vi "Read_Load_Cell_Tensions.vi"(6 "error in (no error)":errorcluster, 7 "Tare Tension":dbl[](array[numeric])=[1.6875269817998764, 0.7228096971601798, 1.962272927280566, 2.6696462364433735, 2.7003690389898463, 3.088938448864716, 1.6430905755314908, 3.0754139877790347, 3.5546581214666455, 3.2737863413382597, 4.727265898547672, 2.6001067118162604, 1.980007529135911, 1.8614502099489874], 8 "sampling freq [Hz]":dbl=1000.0 format="%#_13g", 9 "Refnum in":refnum<k21>="SCI_TenSen") -> (0 "error out":errorcluster={"status"=TRUE, "code"=-200279, "source"="Read_Load_Cell_Tensions.vi<append>\n<B>Property: </B>RelativeTo\n<B>Requested Value: </B>Current Read Position\n\n<B>Property: </B>Offset\n<B>Requested Value: </B>0\n\n<B>Task Name: </B>SCI_TenSen"}, 2 "Measured Cable Tensions":dbl[](array[numeric])=[nan, nan, nan, nan, nan, nan, nan, nan, nan, nan, nan, nan, nan, nan], 3 "Refnum out":refnum<k21>="SCI_TenSen")   [LabVIEW 2024]
uses:
  <vilib>/Analysis/3filter.llb/Filter Passband Type.ctl
  <vilib>/DAQmx/read.llb/DAQmx Read (Analog 2D DBL NChan NSamp).vi
  <vilib>/Analysis/baseanly.llb/Mean (DBL).vi
  <vilib>/DAQmx/miscellaneous.llb/DAQmx Fill In Error Info.vi
  <vilib>/ptbypt/NI_PtbyPt.lvlib
  <vilib>/Analysis/NI_AALBase.lvlib
panel:
  in  "Load Cell Calibration":dbl[][](array[numeric])=[[124.7777, -0.594, 0.0], [124.887, -0.0754, 0.0], [126.3496, 0.0338, 0.0], [126.1641, 0.0078, 0.0], [122.1693, -0.083, 0.0], [125.7362, 0.3615, 0.0], [124.4104, -0.0707, 0.0], [125.885, -0.4858, 0.0], [124.7524, -0.1227, 0.0], [117.4341, 0.7228, 0.0], [124.1327, 0.2733, 0.0], [125.7391, -0.147, 0.0], [125.9788, -0.1556, 0.0], [123.4595, -0.0054, 0.0], [0.0, 0.0, 124.7777]] format="%#_20g"
  in  "Filter Order":i32=2
  in  "cutoff freq [Hz]":dbl=20.0 format="%0.3f"
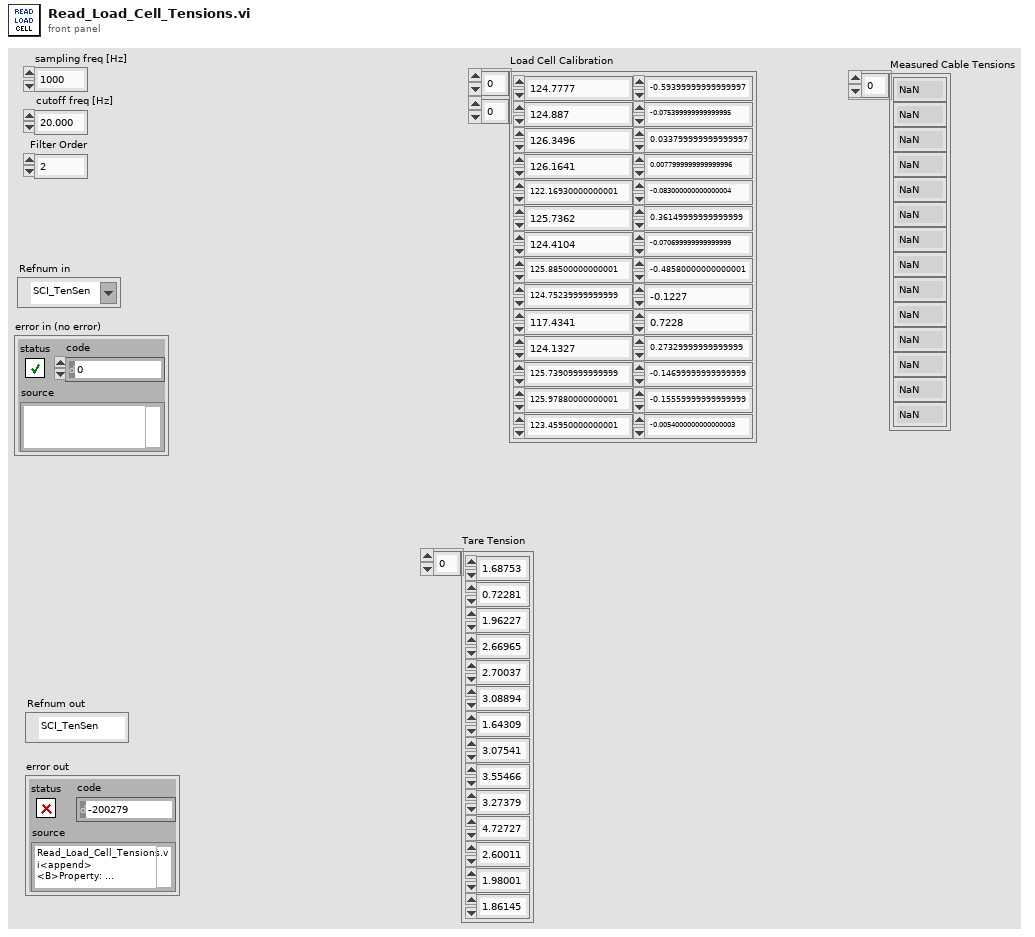
[diagram p1: front panel]
types:
  T1 = typedef "NI_AALBase.lvlib/Filter Passband Type.ctl" = enum32{"Lowpass", "Highpass", "Bandpass", "Bandstop"}
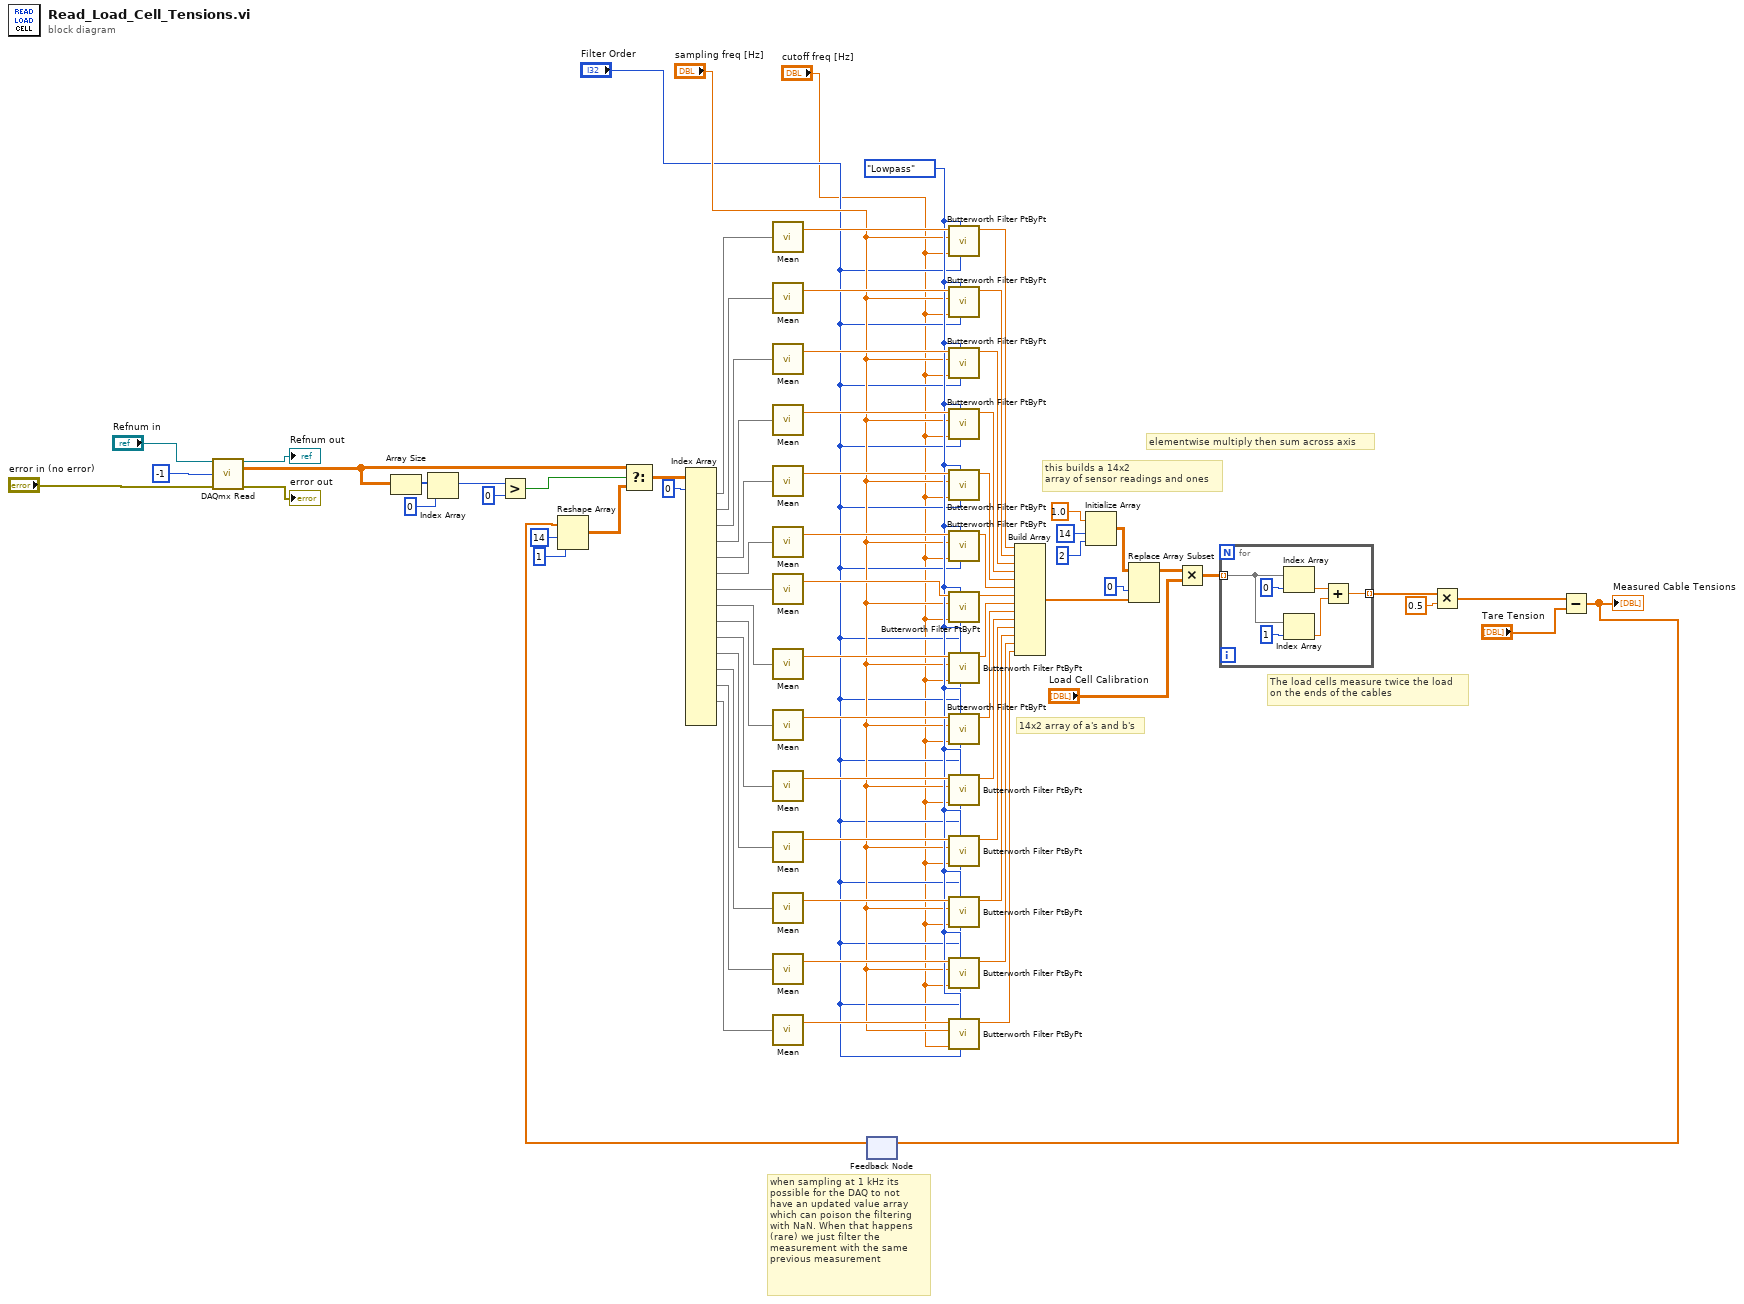
[diagram p0: block diagram]
diagram:
  w14 = Filter_Passband_Type."Lowpass" ("filter type")
  # "when sampling at 1 kHz its \npossible for the DAQ to not\nhave an updated value array\nwhich can poison the filtering\nwith NaN. When that happens\n(rare) we just filter the \nmeasurement with the same\nprevious measurement"
  # "elementwise multiply then sum across axis"
  # "this builds a 14x2\narray of sensor readings and ones"
  # "14x2 array of a's and b's"
  # "The load cells measure twice the load\non the ends of the cables"
  n1 = call-poly <vilib>:"DAQmx Read.vi"("task/channels in"="Refnum in", "number of samples per channel"=-1, "error in"="error in (no error)") -> ("task out"=→"Refnum out":refnum<k21>, "data"=w17:dbl[][], "error out"=→"error out":errorcluster)  [unwired: 10 in]
  n2 = Array Size(array=w17) -> (size(s)=w11:i32[])
  n3 = Index Array(array=w11, index=0) -> (element=w9:i32)
  n4 = Greater?(x=w9, y=0) -> (0:w15:bool)
  n5 = feedback #1() -> (w3:dbl[])  [unwired: 1 in]
  n6 = Reshape Array(w3, 14 ("dimension size"), 1 ("dimension size")) -> (w2:dbl[][])
  n7 = Select(t=w17, s=w15, f=w2) -> (s? t:f=w18:dbl[][])
  n8 = Index Array(array=w18, index (row) #1=0 ("index (row)")) -> (element #1=w57:dbl[], element #2=w68:dbl[], element #3=w67:dbl[], element #4=w66:dbl[], element #5=w65:dbl[], element #6=w64:dbl[], element #7=w63:dbl[], element #8=w60:dbl[], element #9=w48:dbl[], element #10=w47:dbl[], element #11=w46:dbl[], element #12=w45:dbl[], element #13=w44:dbl[], element #14=w43:dbl[])  [unwired: 29 in, 1 out]
  n9 = call-poly <vilib>:"Mean.vi"("X"=w57) -> ("mean"=w56:dbl)  [unwired: 1 out]
  n10 = call-poly <vilib>:"Mean.vi"("X"=w68) -> ("mean"=w74:dbl)  [unwired: 1 out]
  n11 = call-poly <vilib>:"Mean.vi"("X"=w67) -> ("mean"=w73:dbl)  [unwired: 1 out]
  n12 = call-poly <vilib>:"Mean.vi"("X"=w66) -> ("mean"=w72:dbl)  [unwired: 1 out]
  n13 = call-poly <vilib>:"Mean.vi"("X"=w65) -> ("mean"=w71:dbl)  [unwired: 1 out]
  n14 = call-poly <vilib>:"Mean.vi"("X"=w64) -> ("mean"=w70:dbl)  [unwired: 1 out]
  n15 = call-poly <vilib>:"Mean.vi"("X"=w63) -> ("mean"=w69:dbl)  [unwired: 1 out]
  n16 = call-poly <vilib>:"Mean.vi"("X"=w60) -> ("mean"=w59:dbl)  [unwired: 1 out]
  n17 = call-poly <vilib>:"Mean.vi"("X"=w48) -> ("mean"=w42:dbl)  [unwired: 1 out]
  n18 = call-poly <vilib>:"Mean.vi"("X"=w47) -> ("mean"=w41:dbl)  [unwired: 1 out]
  n19 = call-poly <vilib>:"Mean.vi"("X"=w46) -> ("mean"=w40:dbl)  [unwired: 1 out]
  n20 = call-poly <vilib>:"Mean.vi"("X"=w45) -> ("mean"=w39:dbl)  [unwired: 1 out]
  n21 = call-poly <vilib>:"Mean.vi"("X"=w44) -> ("mean"=w38:dbl)  [unwired: 1 out]
  n22 = call-poly <vilib>:"Mean.vi"("X"=w43) -> ("mean"=w37:dbl)  [unwired: 1 out]
  n23 = call <vilib>:"Butterworth Filter PtByPt.vi"("order"="Filter Order", "filter type"=w14, "low cutoff freq: fl"="cutoff freq [Hz]", "sampling freq: fs"="sampling freq [Hz]", "x"=w56) -> ("Filtered x"=w55:dbl)  [unwired: 4 in, 1 out]
  n24 = call <vilib>:"Butterworth Filter PtByPt.vi"("order"="Filter Order", "filter type"=w14, "low cutoff freq: fl"="cutoff freq [Hz]", "sampling freq: fs"="sampling freq [Hz]", "x"=w74) -> ("Filtered x"=w49:dbl)  [unwired: 4 in, 1 out]
  n25 = call <vilib>:"Butterworth Filter PtByPt.vi"("order"="Filter Order", "filter type"=w14, "low cutoff freq: fl"="cutoff freq [Hz]", "sampling freq: fs"="sampling freq [Hz]", "x"=w73) -> ("Filtered x"=w51:dbl)  [unwired: 4 in, 1 out]
  n26 = call <vilib>:"Butterworth Filter PtByPt.vi"("order"="Filter Order", "filter type"=w14, "low cutoff freq: fl"="cutoff freq [Hz]", "sampling freq: fs"="sampling freq [Hz]", "x"=w72) -> ("Filtered x"=w50:dbl)  [unwired: 4 in, 1 out]
  n27 = call <vilib>:"Butterworth Filter PtByPt.vi"("order"="Filter Order", "filter type"=w14, "low cutoff freq: fl"="cutoff freq [Hz]", "sampling freq: fs"="sampling freq [Hz]", "x"=w71) -> ("Filtered x"=w52:dbl)  [unwired: 4 in, 1 out]
  n28 = call <vilib>:"Butterworth Filter PtByPt.vi"("order"="Filter Order", "filter type"=w14, "low cutoff freq: fl"="cutoff freq [Hz]", "sampling freq: fs"="sampling freq [Hz]", "x"=w70) -> ("Filtered x"=w53:dbl)  [unwired: 4 in, 1 out]
  n29 = call <vilib>:"Butterworth Filter PtByPt.vi"("order"="Filter Order", "filter type"=w14, "low cutoff freq: fl"="cutoff freq [Hz]", "sampling freq: fs"="sampling freq [Hz]", "x"=w69) -> ("Filtered x"=w32:dbl)  [unwired: 4 in, 1 out]
  n30 = call <vilib>:"Butterworth Filter PtByPt.vi"("order"="Filter Order", "filter type"=w14, "low cutoff freq: fl"="cutoff freq [Hz]", "sampling freq: fs"="sampling freq [Hz]", "x"=w59) -> ("Filtered x"=w54:dbl)  [unwired: 4 in, 1 out]
  n31 = call <vilib>:"Butterworth Filter PtByPt.vi"("order"="Filter Order", "filter type"=w14, "low cutoff freq: fl"="cutoff freq [Hz]", "sampling freq: fs"="sampling freq [Hz]", "x"=w42) -> ("Filtered x"=w36:dbl)  [unwired: 4 in, 1 out]
  n32 = call <vilib>:"Butterworth Filter PtByPt.vi"("order"="Filter Order", "filter type"=w14, "low cutoff freq: fl"="cutoff freq [Hz]", "sampling freq: fs"="sampling freq [Hz]", "x"=w41) -> ("Filtered x"=w35:dbl)  [unwired: 4 in, 1 out]
  n33 = call <vilib>:"Butterworth Filter PtByPt.vi"("order"="Filter Order", "filter type"=w14, "low cutoff freq: fl"="cutoff freq [Hz]", "sampling freq: fs"="sampling freq [Hz]", "x"=w40) -> ("Filtered x"=w30:dbl)  [unwired: 4 in, 1 out]
  n34 = call <vilib>:"Butterworth Filter PtByPt.vi"("order"="Filter Order", "filter type"=w14, "low cutoff freq: fl"="cutoff freq [Hz]", "sampling freq: fs"="sampling freq [Hz]", "x"=w39) -> ("Filtered x"=w31:dbl)  [unwired: 4 in, 1 out]
  n35 = call <vilib>:"Butterworth Filter PtByPt.vi"("order"="Filter Order", "filter type"=w14, "low cutoff freq: fl"="cutoff freq [Hz]", "sampling freq: fs"="sampling freq [Hz]", "x"=w38) -> ("Filtered x"=w34:dbl)  [unwired: 4 in, 1 out]
  n36 = call <vilib>:"Butterworth Filter PtByPt.vi"("order"="Filter Order", "filter type"=w14, "low cutoff freq: fl"="cutoff freq [Hz]", "sampling freq: fs"="sampling freq [Hz]", "x"=w37) -> ("Filtered x"=w33:dbl)  [unwired: 4 in, 1 out]
  n37 = Build Array(w55, w49, w51, w50, w52, w53, w32, w54, w36, w35, w30, w31, w34, w33) -> (w24:dbl[])
  n38 = Initialize Array(1.0 ("element"), 14 ("dimension size"), 2 ("dimension size")) -> (w25:dbl[][])
  n39 = Replace Array Subset(array=w25, new element=w24, index (col)=0 ("disabled index (col)")) -> (w22:dbl[][])  [unwired: 1 in]
  n40 = Multiply(x=w22, y="Load Cell Calibration") -> (x*y=w20:dbl[][])
  n41 = for {
    tunnel: w20 -> [w83] mode=indexing
    tunnel: [w78] -> w19 mode=indexing
    n42 = Index Array(array=w83, index=0) -> (element=w80:dbl)
    n43 = Index Array(array=w83, index=1) -> (element=w79:dbl)
    n44 = Add(x=w80, y=w79) -> (x+y=w78:dbl)
  }
  n45 = Multiply(x=w19, y=0.5) -> (x*y=w7:dbl[])
  n46 = Subtract(x=w7, y="Tare Tension") -> (x-y=w1:dbl[])
  "Measured Cable Tensions" <- w1
  n47 = feedback-in #1(w1) -> ()
